vi "OP500_BOITE_DIALOGUE_DTC.vi"(0 "Enable":bool=TRUE caption="Activer", 5 "error in (no error)":errorcluster caption="entrée d'erreur (pas d'erreur)") -> (16 "Présence de DTC":bool, 17 "Aucun DTC":bool, 18 "OK":bool, 19 "error out":errorcluster caption="sortie d'erreur")   [LabVIEW 2020]
doc: "Affiche une boîte de dialogue standard qui invite l'utilisateur à entrer des informations, telles qu'un nom d'utilisateur et un mot de passe.\n--------------------\n\nCe VI Express est configuré comme suit :\n\nMessage à afficher à l'utilisateur :Y'a-t-il des DTC restants?\nLes entrées sont : \nCase à cocher : Aucun DTC\nCase à cocher : Présence de DTC"
panel:
  in  "Présence de DTC":bool
  in  "Aucun DTC":bool
  out "String":string="Y'a-t-il des DTC restants?" caption="Chaîne"
  in  "Cancel":bool caption="Annuler"
  in  "OK2":bool
  in  "OK1":bool
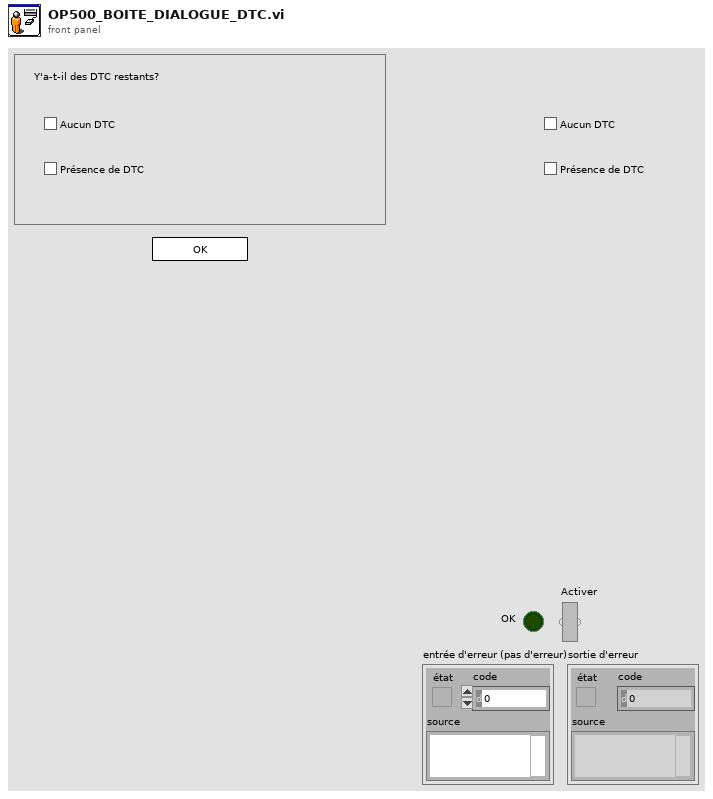
[diagram p1: front panel]
types:
  T1 = cluster{"Input Name":string, "Input Data Type":i32}[]
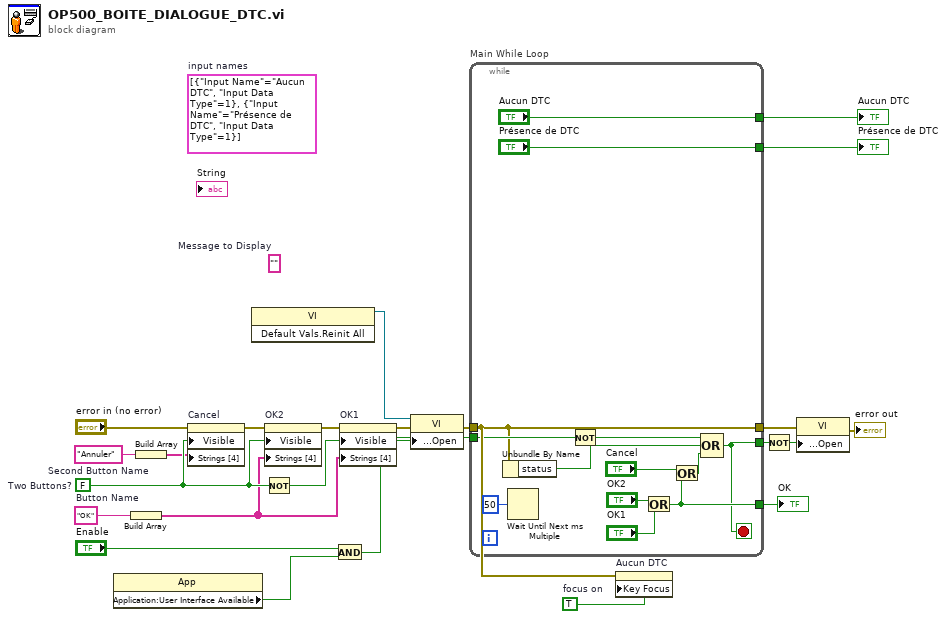
[diagram p0: block diagram]
diagram:
  w2 = TRUE  # focus on
  (unwired) T1 [{"Input Name"="Aucun DTC", "Input Data Type"=1}, {"Input Name"="Présence de DTC", "Input Data Type"=1}]  # input names
  w15 = "Annuler"  # Second Button Name
  w13 = "OK"  # Button Name
  (unwired) ""  # Message to Display
  w23 = FALSE  # Two Buttons?
  n1 = property class="App"() -> ("Application:User Interface Available"=w5:bool)  [unwired: 2 in, 2 out]
  n2 = Build Array(w13) -> (w14:string[])
  n3 = Build Array(w15) -> (w16:string[])
  n4 = property on="Cancel" class="Bool"(error in="error in (no error)", "Visible"=w23, "Strings [4]"=w16) -> (error out=w20:errorcluster)  [unwired: 1 in, 1 out]
  n5 = invoke class="VI" method="Default Vals.Reinit All"() -> (reference out=w4:refnum<vi>)  [unwired: 3 in, 2 out]
  n6 = Not(x=w23) -> (.not. x?=w21:bool)
  n7 = property on="OK2" class="Bool"(error in=w20, "Visible"=w23, "Strings [4]"=w14) -> (error out=w19:errorcluster)  [unwired: 1 in, 1 out]
  n8 = And(x="Enable", y=w5) -> (x .and. y?=w6:bool)
  n9 = property on="OK1" class="Bool"(error in=w19, "Visible"=w21, "Strings [4]"=w14) -> (error out=w12:errorcluster)  [unwired: 1 in, 1 out]
  n10 = property class="VI"(reference=w4, error in=w12, "Front Panel Window:Open"=w6) -> (error out=w11:errorcluster)  [unwired: 1 out]
  n11 = while "Main While Loop" {
    tunnel: [w33] -> w22
    tunnel: w6 -> [w31]
    tunnel: [w29] -> w17
    tunnel: w11 -> [w28]
    tunnel: [w28] -> w9
    tunnel: ["Aucun DTC"] -> w3
    tunnel: ["Présence de DTC"] -> w1
    stop <- w29 stop-if-true
    n12 = Unbundle By Name(w28) -> ("status"=w26:bool)
    n13 = Wait Until Next ms Multiple(millisecond multiple=u32 50) -> ()  [unwired: 1 out]
    n14 = Not(x=w31) -> (.not. x?=w30:bool)
    n15 = Or(x="OK2", y="OK1") -> (x .or. y?=w33:bool)
    n16 = Or(x="Cancel", y=w33) -> (x .or. y?=w27:bool)
    n17 = Compound Arithmetic op=OR(w30, w26, w27) -> (w29:bool)
  }
  "OK" <- w22
  "Aucun DTC" <- w3
  "Présence de DTC" <- w1
  n18 = property on="Aucun DTC" class="Bool (strict)"(error in=w11, "Key Focus"=w2) -> ()  [unwired: 1 in, 2 out]
  n19 = Not(x=w17) -> (.not. x?=w18:bool)
  n20 = property class="VI"(error in=w9, "Front Panel Window:Open"=w18) -> (error out=→"error out":errorcluster)  [unwired: 1 in, 1 out]
